vi "TEST Drop In.vi"(8 "error in (no error)":errorcluster, 10 "Queue Name":string="Main") -> (0 "error out":errorcluster)   [LabVIEW 2011]
doc: "This VI is used to test the functionality of the drop in. However, any VI that has documented controls could also test and utilize the associated drop in.\n\nAAL 9/09"
uses:
  Shared/QDMH Poly VIs/QDMH POLY Enqueue String.vi
panel:
  in  "Test 3":bool
  in  "Test 2":bool
  in  "Test 1":bool
  out "Message Display":string
  in  "Exit":bool
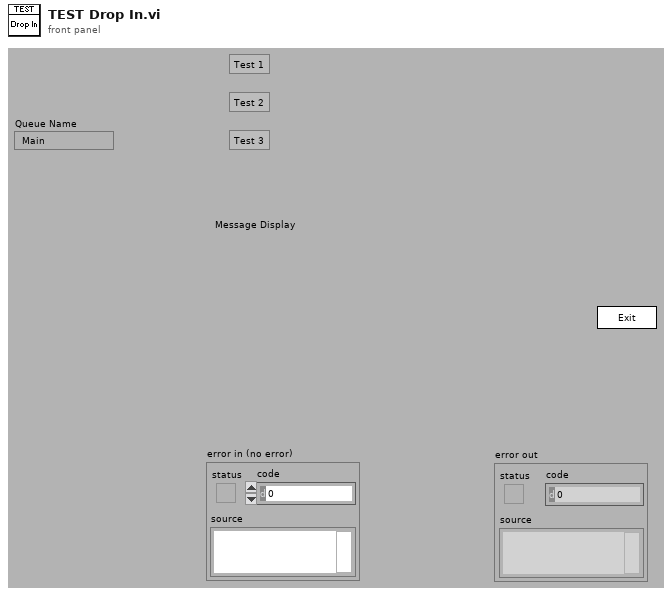
[diagram p1: front panel]
types:
  T1 = cluster{"Operator Name":string, "Current VI's Path":path, "Current VI's  Directory":path, "Queue Names":string[], "# VIs Launched":i32}
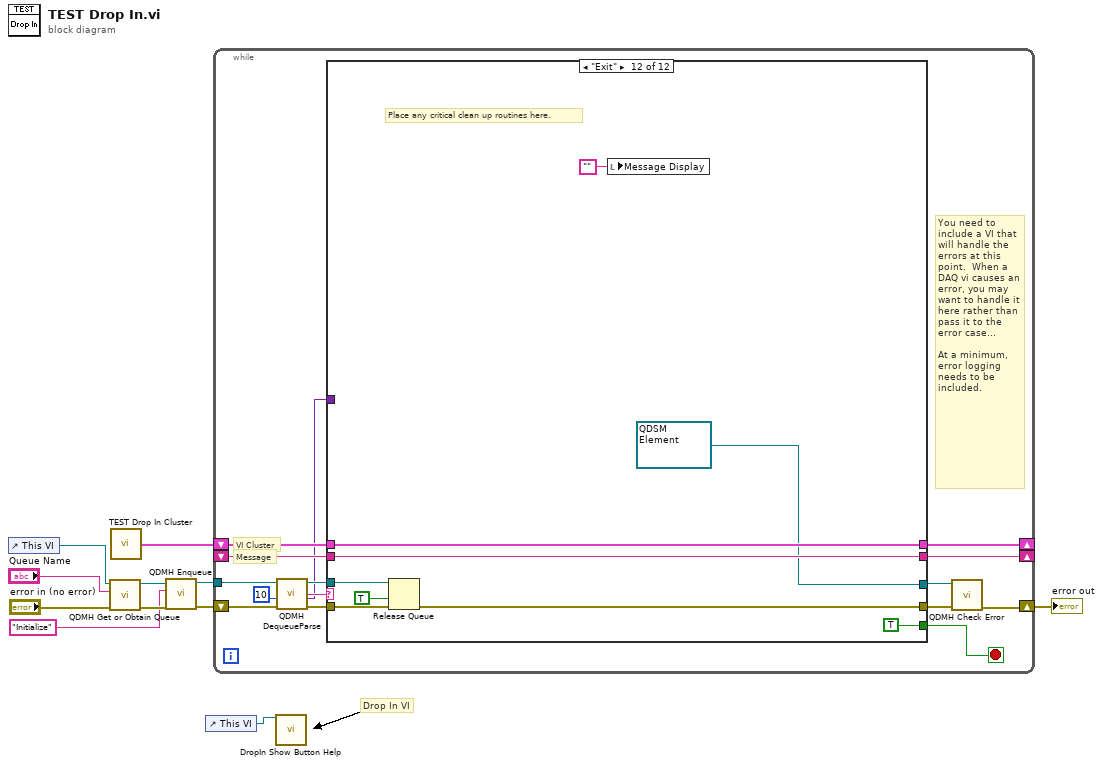
[diagram p0: block diagram]
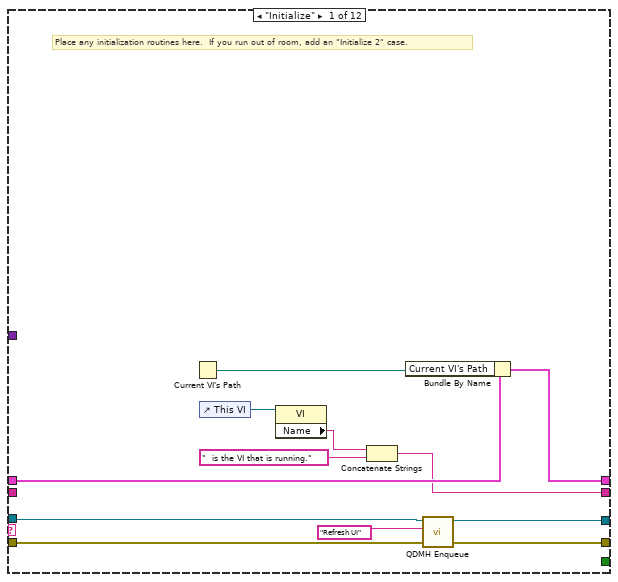
[diagram p2: hidden frame]
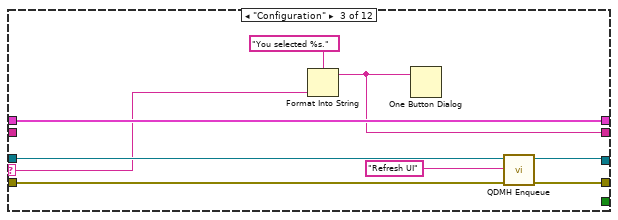
[diagram p4: hidden frame]
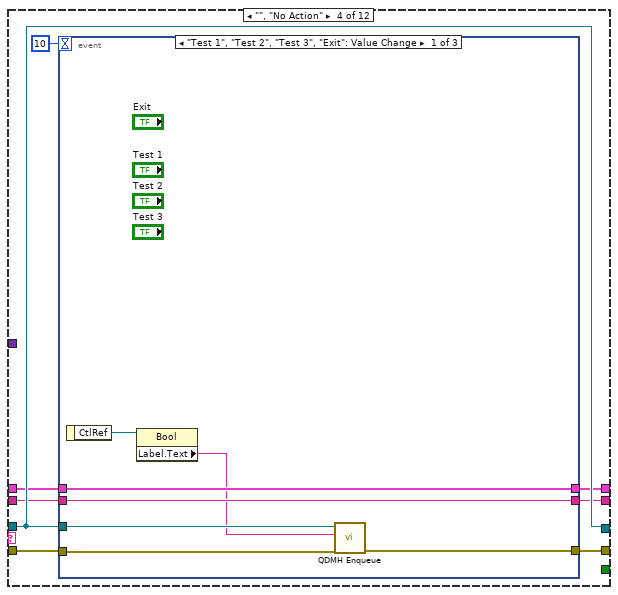
[diagram p5: hidden frame]
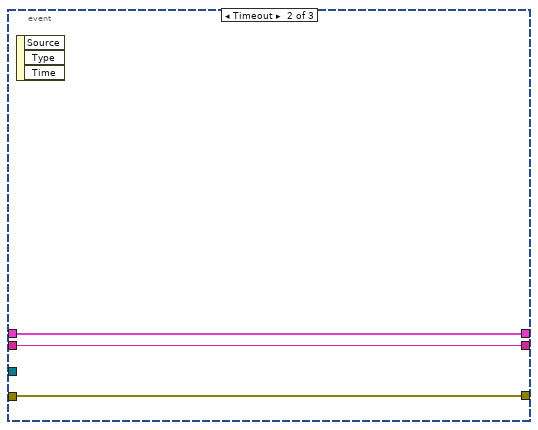
[diagram p6: hidden frame]
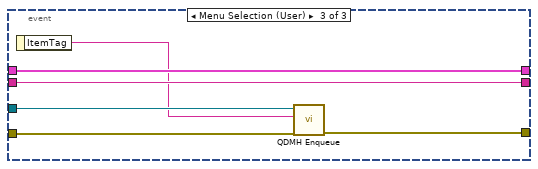
[diagram p7: hidden frame]
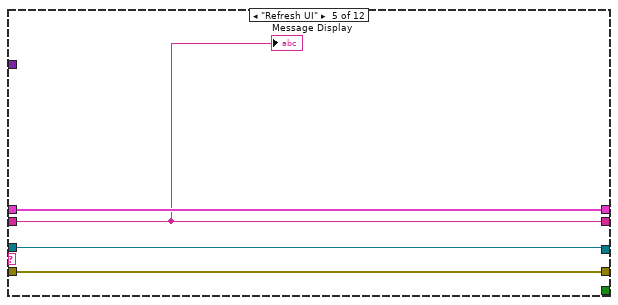
[diagram p8: hidden frame]
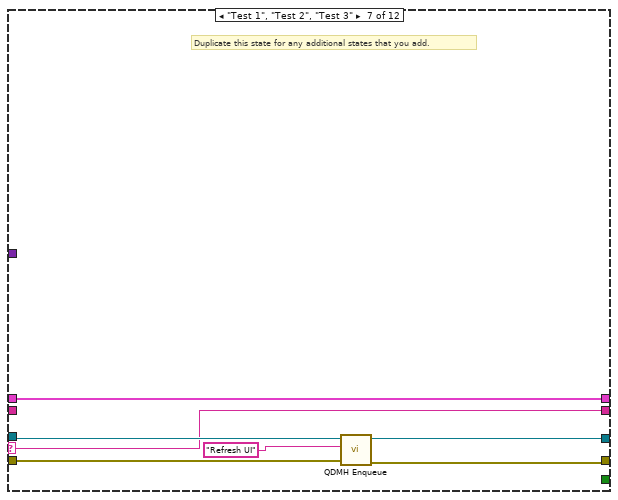
[diagram p10: hidden frame]
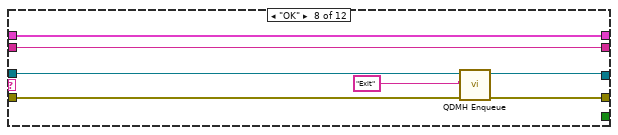
[diagram p11: hidden frame]
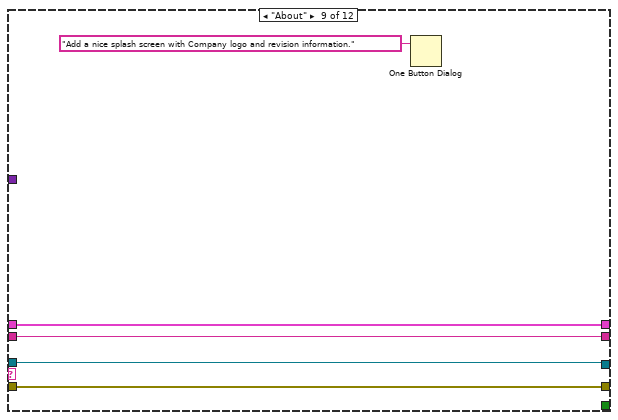
[diagram p12: hidden frame]
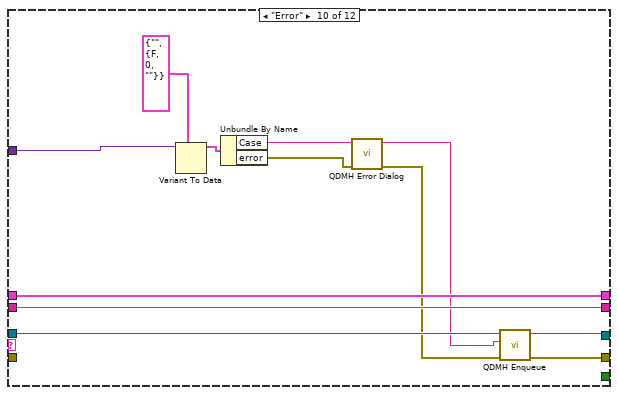
[diagram p13: hidden frame]
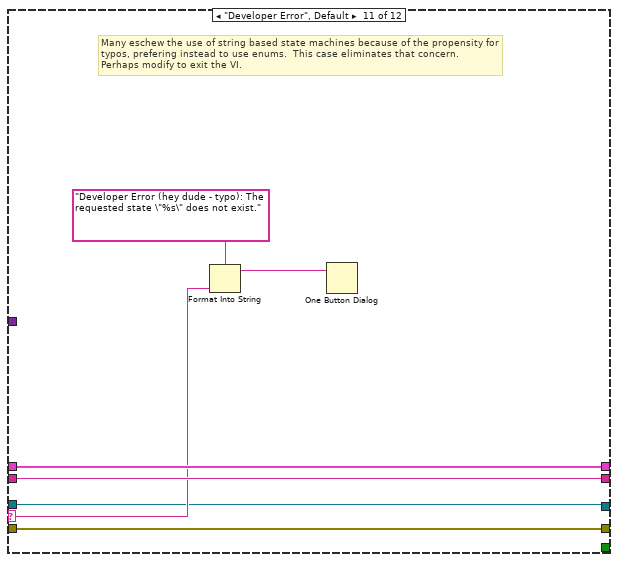
[diagram p14: hidden frame]
diagram:
  # "Drop In VI"
  n1 = control-ref of="This VI"() -> (w3:refnum<vi>)
  n2 = call "QDMH Get or Obtain Queue.vi"("error in (no error)"="error in (no error)", "Queue Name"="Queue Name", "VI Refnum"=w3) -> ("error out"=w7:errorcluster, "queue out"=w10:refnum<queue>)  [unwired: 7 out]
  n3 = call "TEST Drop In Cluster.vi"() -> ("Cluster"=w9:T1)
  n4 = call-poly "QDMH Enqueue.vi"("error in (no error)"=w7, "State"="Initialize" ("element"), "queue"=w10) -> ("error out"=w8:errorcluster, "queue out"=w11:refnum<queue>)  [unwired: 7 out]
  n5 = control-ref of="This VI"() -> (w1:refnum<vi>)
  n6 = while {
    tunnel: w11 -> [w21]
    shift-left: w9 -> [w22]
    shift-right: [w23] -> _
    shift-left: _ -> [w24]
    shift-right: [w25] -> _
    shift-right: [w15] -> w5
    shift-left: w8 -> [w16]
    stop <- w26 stop-if-true
    # "VI Cluster"
    # "Message"
    # "You need to include a VI that will handle the errors at this point.  When a DAQ vi causes an error, you may want to handle it here rather than pass it to the error case...\n\nAt a minimum,\nerror logging\nneeds to be \nincluded."
    n7 = call "QDMH DequeueParse.vi"("error in (no error)"=w16, "Timeout"=10 ("ms timeout (-1)"), "queue"=w21) -> ("error out"=w18:errorcluster, "Variant Data"=w12:variant, "State"=w17:string, "queue out"=w19:refnum<queue>)  [unwired: 5 out]
    n8 = case shown="\"Exit\"" w17 {
      selector: w17 -> [_ _ w47 _ _ _ w86 _ _ _ w118 _]
      tunnel: w19 -> [w33 w39 w49 w59 w76 w80 w88 w97 w98 w112 w115 w127]
      tunnel: [_ _ _ _ _ _ _ _ _ _ _ TRUE] -> w26
      tunnel: [w31 w42 w48 w52 w78 w83 w86 w96 w102 w114 w121 w129] -> w25
      tunnel: w24 -> [_ w42 _ w53 w78 w83 _ w96 w102 w114 w121 w129]
      tunnel: [w37 w41 w51 w54 w79 w82 w90 w95 w101 w113 w120 w124] -> w23
      tunnel: w22 -> [w38 w41 w51 w55 w79 w82 w90 w95 w101 w113 w120 w124]
      tunnel: w18 -> [w35 w40 w46 w58 w77 w81 w89 w94 w99 _ w117 w126]
      tunnel: [w34 w40 w45 w57 w77 w81 w87 w93 w99 w111 w117 w123] -> w14
      tunnel: [w27 w39 w43 w59 w76 w80 w84 w92 w98 w110 w115 refnum<queue> refnum ("queue out")] -> w13
      tunnel: w12 -> [_ _ _ _ _ _ _ _ _ w105 _ _]
      frame "Initialize" {
        # "Place any initialization routines here.  If you run out of room, add an \"Initialize 2\" case."
        n9 = Current VI's Path() -> (path=w36:path)
        n10 = control-ref of="This VI"() -> (w30:refnum<vi>)
        n11 = property class="VI"(reference=w30) -> ("Name"=w29:string)  [unwired: 1 in, 2 out]
        n12 = Concatenate Strings(w29, "  is the VI that is running." ("string")) -> (w31:string)
        n13 = Bundle By Name(cluster=w38, "Current VI's Path"=w36) -> (w37:T1)
        n14 = call-poly "QDMH Enqueue.vi"("error in (no error)"=w35, "State"="Refresh UI" ("New State"), "queue"=w33) -> ("error out"=w34:errorcluster, "queue out"=w27:refnum<queue>)  [unwired: 7 out]
      }
      frame "Re-Initialize" {
        # "This case includes initialization functionality that may need to run again during the course of the VI"
      }
      frame "Configuration" {
        n15 = Format Into String(format string="You selected %s." ("Format String"), w47) -> (resulting string=w48:string)  [unwired: 2 in, 1 out]
        n16 = One Button Dialog(message=w48) -> ()  [unwired: 2 out]
        n17 = call-poly "QDMH Enqueue.vi"("error in (no error)"=w46, "State"="Refresh UI" ("New State"), "queue"=w49) -> ("error out"=w45:errorcluster, "queue out"=w43:refnum<queue>)  [unwired: 7 out]
      }
      frame "", "No Action" {
        n18 = event shown="[0] \"Test 1\", \"Test 2\", \"Test 3\", \"Exit\": Value Change" {
          selector: _ -> [_ _ _]
          dyn-events: _ -> [_ _ _]
          timeout: 10 -> [_ _ _]
          tunnel: w59 -> [w65 _ w75]
          tunnel: [w64 w69 w73] -> w57
          tunnel: w58 -> [w63 w69 w74]
          tunnel: w55 -> [w62 w68 w72]
          tunnel: [w62 w68 w72] -> w54
          tunnel: w53 -> [w61 w67 w71]
          tunnel: [w61 w67 w71] -> w52
          event "Test 1", "Test 2", "Test 3", "Exit": Value Change {
            n19 = event-data() -> ("CtlRef"=w66:refnum<vi>)  [unwired: 1 out]
            n20 = property class="Bool"(reference=w66) -> ("Label.Text"=w60:string)  [unwired: 1 in, 2 out]
            n21 = call-poly "QDMH Enqueue.vi"("error in (no error)"=w63, "State"=w60, "queue"=w65) -> ("error out"=w64:errorcluster)  [unwired: 8 out]
          }
          event Timeout {
            n22 = event-data() -> ()  [unwired: 4 out]
          }
          event Menu Selection (User) {
            n23 = event-data() -> ("ItemTag"=w70:string)  [unwired: 1 out]
            n24 = call-poly "QDMH Enqueue.vi"("error in (no error)"=w74, "State"=w70, "queue"=w75) -> ("error out"=w73:errorcluster)  [unwired: 8 out]
          }
        }
      }
      frame "Refresh UI" {
        "Message Display" <- w78
      }
      frame "<add states as needed>" {
        # "Duplicate this state for any additional states that you add."
      }
      frame "Test 1", "Test 2", "Test 3" {
        # "Duplicate this state for any additional states that you add."
        n25 = call-poly "QDMH Enqueue.vi"("error in (no error)"=w89, "State"="Refresh UI" ("element"), "queue"=w88) -> ("error out"=w87:errorcluster, "queue out"=w84:refnum<queue>)  [unwired: 7 out]
      }
      frame "OK" {
        n26 = call-poly "QDMH Enqueue.vi"("error in (no error)"=w94, "State"="Exit" ("New State"), "queue"=w97) -> ("error out"=w93:errorcluster, "queue out"=w92:refnum<queue>)  [unwired: 7 out]
      }
      frame "About" {
        n27 = One Button Dialog(message="Add a nice splash screen with Company logo and revision information.") -> ()  [unwired: 2 out]
      }
      frame "Error" {
        n28 = Variant To Data(type=cluster{"Case":string, "error":errorcluster} {"Case"="", "error"={"status"=FALSE, "code"=0, "source"=""}} ("QDSM Element"), Variant=w105) -> (data=w107:cluster{"Case":string, "error":errorcluster})  [unwired: 1 in, 1 out]
        n29 = Unbundle By Name(w107) -> ("Case"=w108:string, "error"=w109:errorcluster)
        n30 = call "QDMH Error Dialog.vi"("error"=w109, "Case Error Occured"=w108) -> ("error out (no error)"=w104:errorcluster, "Case to Execute"=w103:string)  [unwired: 8 out]
        n31 = call-poly "QDMH Enqueue.vi"("error in (no error)"=w104, "State"=w103, "queue"=w112) -> ("error out"=w111:errorcluster, "queue out"=w110:refnum<queue>)  [unwired: 7 out]
      }
      frame "Developer Error", Default {
        # "Many eschew the use of string based state machines because of the propensity for\ntypos, prefering instead to use enums.  This case eliminates that concern.\nPerhaps modify to exit the VI."
        n32 = Format Into String(format string="Developer Error (hey dude - typo): The requested state \"%s\" does not exist." ("message"), w118) -> (resulting string=w116:string)  [unwired: 2 in, 1 out]
        n33 = One Button Dialog(message=w116) -> ()  [unwired: 2 out]
      }
      frame "Exit" {
        # "Place any critical clean up routines here."
        n34 = Release Queue(queue=w127, force destroy? (F)=TRUE, error in (no error)=w126) -> (error out=w123:errorcluster)  [unwired: 2 out]
        n35 = local write "Message Display"("") -> ()
      }
    }
    n36 = call "QDMH Check Error.vi"("error in (no error)"=w14, "queue"=w13) -> ("error out"=w15:errorcluster)  [unwired: 2 in, 7 out]
  }
  "error out" <- w5
  n37 = call "DropIn Show Button Help.vi"("VI Refnum"=w1) -> ()  [unwired: 14 in, 1 out]
